vi "RESTful VIType To Text.vi"(1 "Service VI Type":T1) -> (0 "Text":string)   [LabVIEW 2020]
uses:
  <vilib>/AppBuilder/AB_Classes/Source/RESTfulVI/Configure_RESTfulVI/AB_RESTful_VIType.ctl
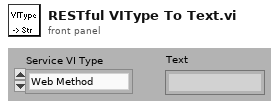
[diagram p1: front panel]
types:
  T1 = typedef "AB_RESTful_VIType.ctl" = enum32{"Web Method", "Auxiliary", "eng_Internal", "eng_Content"}
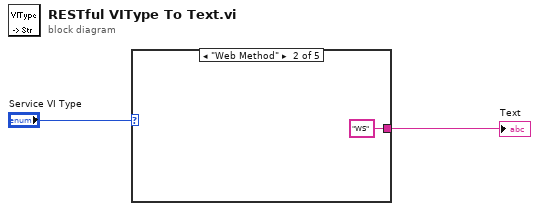
[diagram p0: block diagram]
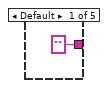
[diagram p2: hidden frame]
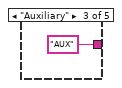
[diagram p3: hidden frame]
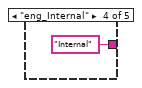
[diagram p4: hidden frame]
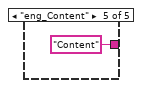
[diagram p5: hidden frame]
diagram:
  n1 = case shown="\"Web Method\"" "Service VI Type" {
    tunnel: ["" ("Boolean Text") "WS" ("Boolean Text") "AUX" ("Boolean Text") "Internal" ("Boolean Text") "Content" ("Boolean Text")] -> w2
    frame Default {
    }
    frame "Web Method" {
    }
    frame "Auxiliary" {
    }
    frame "eng_Internal" {
    }
    frame "eng_Content" {
    }
  }
  "Text" <- w2
